vi "Device Clear.vi"(8 "error in":errorcluster, 11 "VISA resource name":refnum<visa-resource-name>) -> (0 "error out":errorcluster, 3 "VISA resource name out":refnum<visa-resource-name>)   [LabVIEW 2019, in "Andeen-Hagerling 2700.lvlib"]
doc: "Issue a Device Clear command to the bridge. Immediately aborts execution of any command or macro. The bridge is left in a state that should accept a new command."
uses:
  Andeen-Hagerling 2700.lvlib
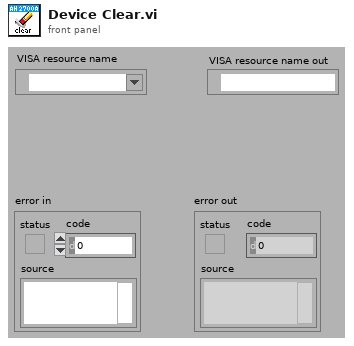
[diagram p1: front panel]
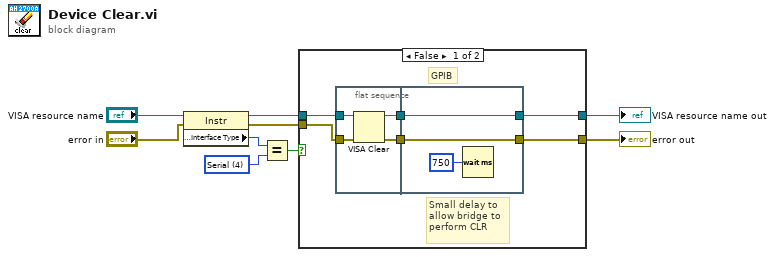
[diagram p0: block diagram]
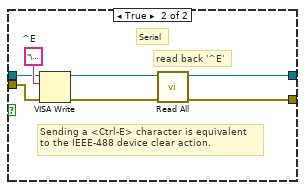
[diagram p2: hidden frame]
diagram:
  w5 = u16 4 items=["GPIB"=1, "VXI"=2, "GPIB-VXI"=3, "Serial"=4, "PXI"=5, "TCPIP"=6, "USB"=7] ("Interface Information:Interface Type")
  n1 = property on="Property Node" class="Instr"(reference="VISA resource name", error in="error in") -> (reference out=w9:refnum<visa-resource-name>, error out=w7:errorcluster, "Interface Information:Interface Type"=w6:u16)
  n2 = Equal?(x=w6, y=w5) -> (x = y?=w8:bool)
  n3 = case shown="False" w8 {
    tunnel: w7 -> [w12 w27]
    tunnel: [w14 w25] -> w3
    tunnel: [w13 w23] -> w4
    tunnel: w9 -> [w15 w28]
    frame False {
      # "Small delay to \nallow bridge to\nperform CLR"
      # "GPIB"
      n4 = flat-sequence {
        tunnel: w15 -> [w19]
        tunnel: w12 -> [w16]
        tunnel: [w18] -> w11
        tunnel: [w17] -> w10
        tunnel: [w21] -> w13
        tunnel: [w22] -> w14
        tunnel: w11 -> [w22]
        tunnel: w10 -> [w21]
        frame #0 {
          n5 = VISA Clear(VISA resource name=w19, error in (no error)=w16) -> (VISA resource name out=w18:refnum<visa-resource-name>, error out=w17:errorcluster)
        }
        frame #1 {
          n6 = Wait (ms)(milliseconds to wait=u32 750) -> ()  [unwired: 1 out]
        }
      }
    }
    frame True {
      w29 = "\u0005"  # ^E
      # "read back '^E'"
      # "Sending a <Ctrl-E> character is equivalent\nto the IEEE-488 device clear action."
      # "Serial"
      n7 = VISA Write(VISA resource name=w28, write buffer=w29, error in (no error)=w27) -> (VISA resource name out=w26:refnum<visa-resource-name>, error out=w24:errorcluster)  [unwired: 1 out]
      n8 = call "Read All.vi"("error in"=w24, "VISA resource name"=w26) -> ("error out"=w23:errorcluster, "VISA resource name out"=w25:refnum<visa-resource-name>)  [unwired: 6 in, 2 out]
    }
  }
  "VISA resource name out" <- w3
  "error out" <- w4
